vi "Is UI.vi"(8 "error in (no error)":errorcluster, 11 "LVClassLibrary in":refnum<vi>) -> (0 "error out":errorcluster, 2 "UI":bool, 3 "LVClassLibrary out":refnum<vi>)   [LabVIEW 2019, in "ProjectItem.lvclass"]
uses:
  ProjectItem.lvclass
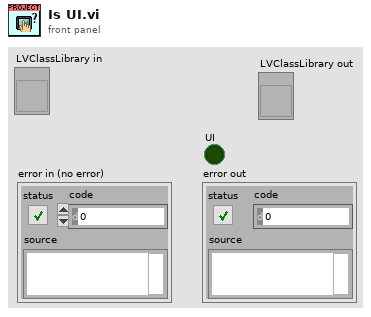
[diagram p1: front panel]
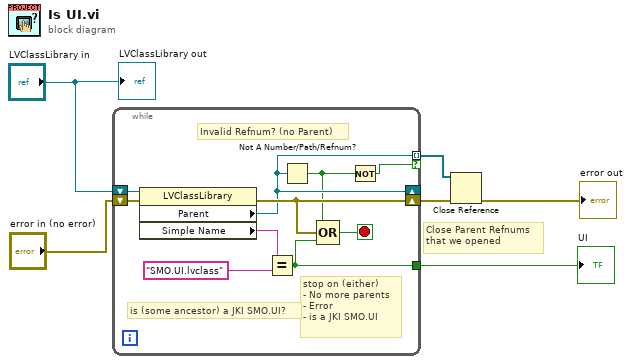
[diagram p0: block diagram]
diagram:
  # "Close Parent Refnums\nthat we opened"
  n1 = while {
    shift-right: [w10] -> _
    shift-left: "LVClassLibrary in" -> [w16]
    tunnel: [w10] -> w3 mode=indexing if=w8
    shift-right: [w11] -> w2
    shift-left: "error in (no error)" -> [w15]
    tunnel: [w13] -> w1
    stop <- w12 stop-if-true
    # "stop on (either)\n- No more parents\n- Error\n- is a JKI SMO.UI"
    # "is (some ancestor) a JKI SMO.UI?"
    # "Invalid Refnum? (no Parent)"
    n2 = property class="LVClassLibrary"(reference=w16, error in=w15) -> (error out=w11:errorcluster, "Parent"=w10:refnum<vi>, "Simple Name"=w7:string)  [unwired: 1 out]
    n3 = Equal?(x=w7, y="SMO.UI.lvclass") -> (x = y?=w13:bool)
    n4 = Not A Number/Path/Refnum?(number/path/refnum=w10) -> (NaN/Path/Refnum?=w9:bool)
    n5 = Compound Arithmetic op=OR(w9, w11, w13) -> (w12:bool)
    n6 = Not(x=w9) -> (.not. x?=w8:bool)
  }
  "UI" <- w1
  n7 = Close Reference(reference=w3, error in (no error)=w2) -> (error out=→"error out":errorcluster)
  "LVClassLibrary out" <- "LVClassLibrary in"
